vi "GE 5565PIORC.Round Up to Nearest 8.vi"(11 "value":u32 format="%08x") -> (3 "aligned value":u32 format="%08x")   [LabVIEW 2024, in "GE 5565PIORC.lvclass"]
uses:
  GE 5565PIORC.lvclass
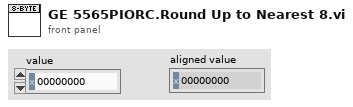
[diagram p1: front panel]
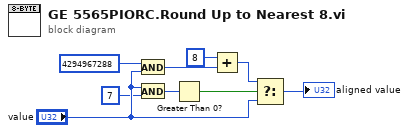
[diagram p0: block diagram]
diagram:
  n1 = And(x=u32 4294967288, y="value") -> (x .and. y?=w7:u32)
  n2 = And(x="value", y=u32 7 ("x")) -> (x .and. y?=w9:u32)
  n3 = Greater Than 0?(x=w9) -> (x > 0?=w8:bool)
  n4 = Add(x=u32 8, y=w7) -> (x+y=w5:u32)
  n5 = Select(t=w5, s=w8, f="value") -> (s? t:f=→"aligned value":u32)
